vi "PCO_GetRecordingState.vi"(8 "error in (no error)":errorcluster {"code" format="%x"}, 11 "ph":u64) -> (0 "error out":errorcluster {"code" format="%x"}, 1 "wRecState":u16(ring) items=["stop", "run"], 2 "ErrorMessage":i32 format="%x", 3 "ph out":u64)   [LabVIEW 2019, in "SDK.lvlib" / "RecordingControl.lvlib"]
doc: "<b>Description:</b>\nThis function returns the current Recording State of the camera.\n\nThe Recording State can change from [run] to [stop] through:\n• Call to function PCO_SetRecordingState [stop]\n• PCO_SetStorageMode is [recorder], PCO_SetRecorderSubmode is [sequence] and active \n segment is full\n• PCO_SetStorageMode is [recorder], PCO_SetRecorderSubmode is [ring buffer], \n PCO_SetRecordStopEvent is [on] and the given number of images is recorded.\n\n<b>Supported camera type:</b>\nAll cameras\n\n<b>Descriptor dependency:</b>\nNone"
uses:
  RecordingControl.lvlib
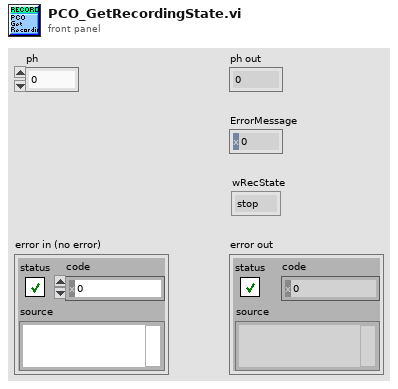
[diagram p1: front panel]
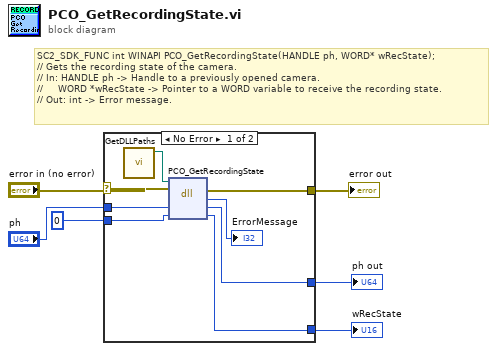
[diagram p0: block diagram]
diagram:
  # "SC2_SDK_FUNC int WINAPI PCO_GetRecordingState(HANDLE ph, WORD* wRecState);\n// Gets the recording state of the camera.\n// In: HANDLE ph -> Handle to a previously opened camera.\n//     WORD *wRecState -> Pointer to a WORD variable to receive the recording state.\n// Out: int -> Error message."
  n1 = case shown="No Error" "error in (no error)" {
    selector: "error in (no error)" -> [w8 w17]
    tunnel: "ph" -> [w13 w16]
    tunnel: [w12 w16] -> w5
    tunnel: u16 0 ("wRecState") -> [w11 w15]
    tunnel: [w10 w15] -> w3
    tunnel: [w9 w17] -> w2
    frame No Error {
      n2 = call "GetDLLPaths.vi"() -> ("SC2_Cam_Path"=w7:path)  [unwired: 9 in, 2 out]
      n3 = dll-call lib="?" fn="PCO_GetRecordingState"(path in=w7, error in=w8, "ph"=w13, "wRecState"=w11) -> (error out=w9:errorcluster, "return type"=→"ErrorMessage":i32, "ph"=w12:u64, "wRecState"=w10:u16)  [unwired: 1 in, 1 out]
    }
    frame Error {
    }
  }
  "ph out" <- w5
  "wRecState" <- w3
  "error out" <- w2
